vi "full_rt_layer.vi"() -> ()   [LabVIEW 2014]
uses:
  <vilib>/LabVIEW Targets/FPGA/cRIO/cRIO-9505/controls.llb/_nicrio_cRIO-9505_DriveStatus.ctl
  <vilib>/FPGAPlugInAG/cRIO-9074/niLvFpga_Open_cRIO-9074.vi
  <vilib>/Utility/error.llb/Error Cluster From Error Code.vi
  <vilib>/rvi/errors/niLvFpgaAdjustHostInterfaceError.vi
  <vilib>/FPGAPlugInAG/cRIO-9074/niLvFpga_Close_cRIO-9074.vi
  <vilib>/rvi/interface/nirviOpenFPGA/nirviOpenFPGA.xnode
  FPGA Bitfiles/MotorLabAProject_FPGATarget_fullfpgalayer_LolEBNhdJec.lvbitx
  full_fpga_layer.vi
  <vilib>/rvi/interface/nirviReadWriteControl/nirviReadWriteControl.xnode
  <vilib>/rvi/interface/nirviCloseFPGA/nirviCloseFPGA.xnode
  NiFpgaLv.dll
panel:
  out "PWM Current  Command":i16
  in  "number":i32
  out "Analog PID Scaled Output":fxp<+/-,34,17>
  in  "Reset Analog Counter":bool
  out "Set Point in Counts":dbl
  out "Waveform Chart 2":cluster{dbl, i32}(graph)
  out "Stepper Current (Steps)":i32
  out "Stepper Steps to move":i32
  in  "Reset Stepper Counter":bool
  out "PWM Angular Position":dbl
  out "Pot Angular \nPosition (deg)":fxp<+/-,33,11>
  out "error out":errorcluster
  in  "Position Loop  Rate (usec)":u16=250
  in  "Position Error Limit":i16=32767
  out "Position Error Read":i16
  out "Position Error Status":bool
  out "Encoder Position":i32
  in  "Reset Encoder Position":bool
  in  "stop":bool
  out "Drive Status":T1=enum."Disabled"
  out "Waveform Chart":cluster{i64, "PWM Encoder Position":i32}(graph)
  # "PWM SERVO"
  # "USE ESTOP!"
  # "ANALOG SERVO"
  # "STEPPER"
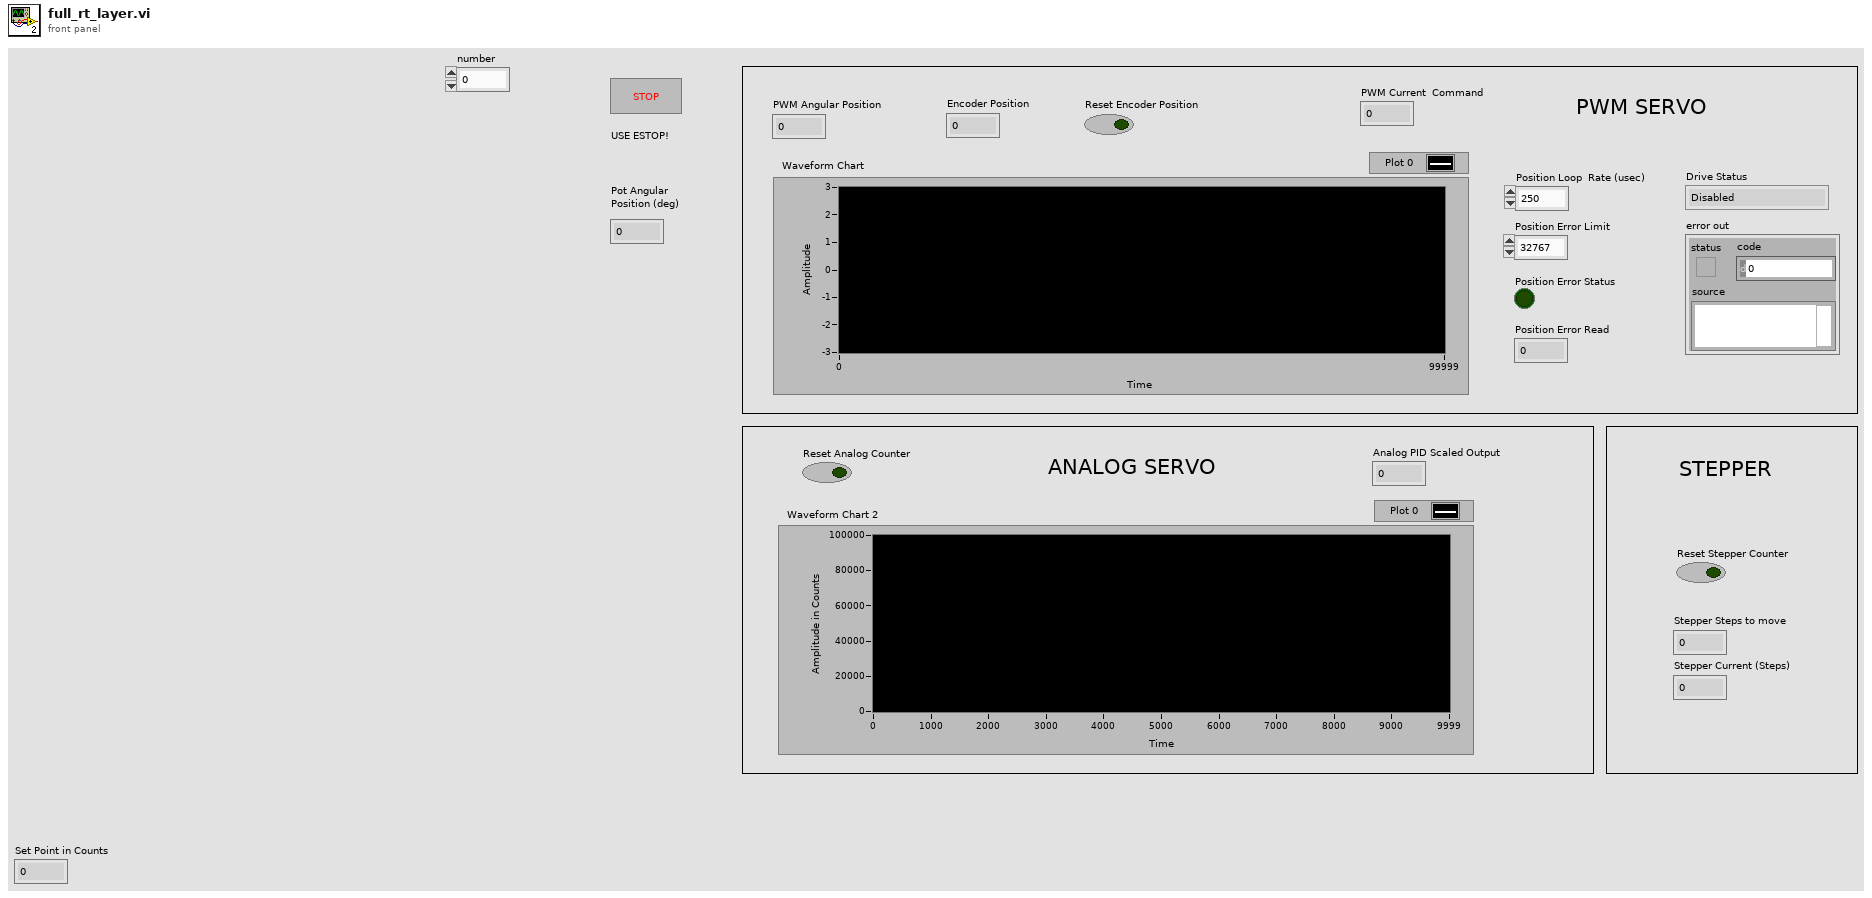
[diagram p1: front panel]
types:
  T1 = typedef "_nicrio_cRIO-9505_DriveStatus.ctl" = enum8{"Enabled", "Disabled", "Disabled by Drive Fault", "Disabled by Temp. Fault", "Disabled by E-Stop", "Unknown"}
  T2 = cluster{"Kp":i16, "Kd":i16, "Ki":i16, "ILim":i16, "Vff":i16, "Vff":i16, "Vff":i16, "Td":i16}
  T3 = cluster{dbl, "Analog Position  Feedback (Counts)":i32}
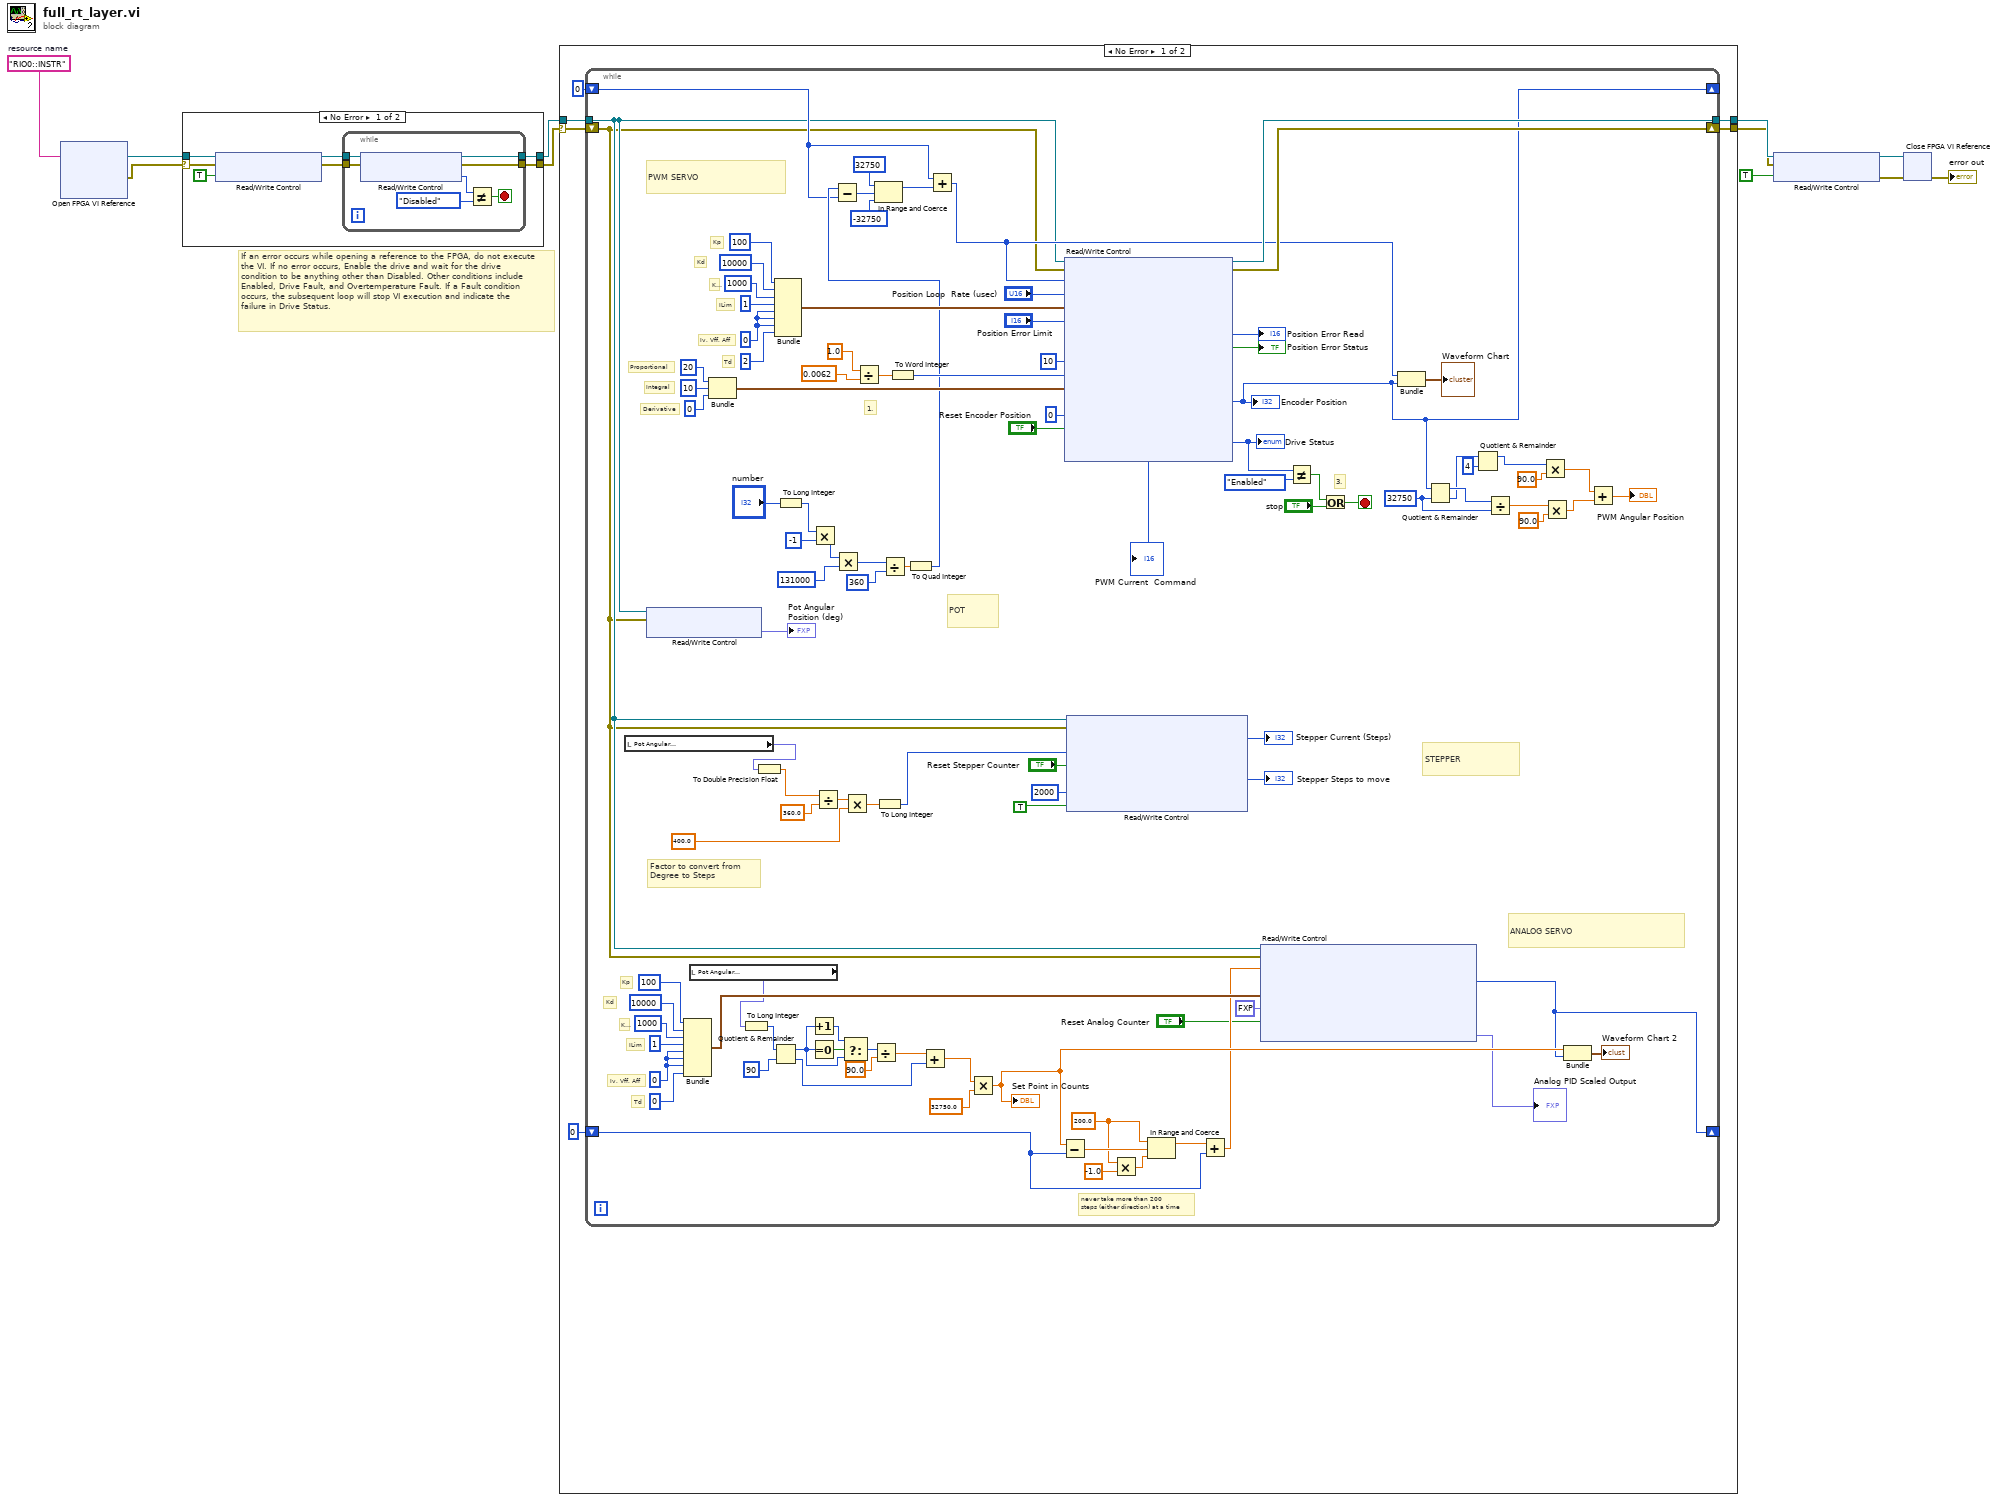
[diagram p0: block diagram]
diagram:
  w2 = "RIO0::INSTR"  # resource name
  # "If an error occurs while opening a reference to the FPGA, do not execute the VI. If no error occurs, Enable the drive and wait for the drive condition to be anything other than Disabled. Other conditions include Enabled, Drive Fault, and Overtemperature Fault. If a Fault condition occurs, the subsequent loop will stop VI execution and indicate the failure in Drive Status."
  n1 = xnode "Open FPGA VI Reference"("resource name"=w2) -> ("FPGA VI Reference Out"=w5:refnum<k20>, "error out"=w4:errorcluster)  [unwired: 1 in]
  n2 = case shown="No Error" w4 {
    selector: w4 -> [w13 w26]
    tunnel: w5 -> [w16 w27]
    tunnel: [w18 w27] -> w6
    tunnel: [w17 w26] -> w3
    frame No Error {
      n3 = xnode "Read/Write Control"("FPGA VI Reference In"=w16, "error in"=w13, "PWM  Enable Drive"=TRUE ("Enable Drive")) -> ("FPGA VI Reference Out"=w15:refnum<k20>, "error out"=w14:errorcluster)
      n4 = while {
        tunnel: [w25] -> w18
        tunnel: [w21] -> w17
        tunnel: w15 -> [w20]
        tunnel: w14 -> [w19]
        stop <- w22 stop-if-true
        n5 = xnode "Read/Write Control"("FPGA VI Reference In"=w20, "error in"=w19) -> ("FPGA VI Reference Out"=w25:refnum<k20>, "error out"=w21:errorcluster, "PWM Drive Status"=w24:T1)
        n6 = Not Equal?(x=w24, y=_nicrio_cRIO-9505_DriveStatus."Disabled") -> (x != y?=w22:bool)
      }
    }
    frame Error {
      # "Error occurred. Do not run."
    }
  }
  n7 = case shown="No Error" w3 {
    selector: w3 -> [w30 w139]
    tunnel: w6 -> [w33 w140]
    tunnel: [w32 w140] -> w11
    tunnel: [w31 w139] -> w10
    frame No Error {
      n8 = while {
        tunnel: w33 -> [w39]
        tunnel: [w134] -> w32
        shift-right: [w110] -> w31
        shift-left: w30 -> [w38]
        shift-right: [w89] -> _
        shift-left: 0 -> [w87]
        shift-right: [w42] -> _
        shift-left: 0 -> [w57]
        stop <- w111 stop-if-true
        w47 = 200.0
        w67 = i16 0 ("Vff")
        w108 = 32750 ("y")
        w120 = i16 0 ("Vff")
        # "never take more than 200 \nsteps (either direction) at a time"
        # "ANALOG SERVO"
        # "STEPPER"
        # "POT"
        # "Td"
        # "Iv, Vff, Aff"
        # "ILim"
        # "Ki"
        # "Kd"
        # "Kp"
        # "Factor to convert from \nDegree to Steps"
        # "PWM SERVO"
        # "Derivative"
        # "Integral"
        # "Proportional"
        # "Td"
        # "Iv, Vff, Aff"
        # "ILim"
        # "Ki"
        # "Kd"
        # "Kp"
        # "3."
        # "1."
        n9 = local read "Pot Angular \nPosition (deg)"() -> (w37:fxp<+/-,33,11>)
        n10 = xnode "Read/Write Control"("FPGA VI Reference In"=w39, "error in"=w38) -> ("Pot Angular Position"=→"Pot Angular \nPosition (deg)":fxp<+/-,33,11>)  [unwired: 2 out]
        n11 = Bundle("Kp"=i16 100, "Kd"=i16 10000, "Ki"=i16 1000, "ILim"=i16 1, "Vff"=w67, "Vff"=w67, "Vff"=w67, "Td"=i16 0) -> (w65:T2)  [unwired: 1 in]
        n12 = local read "Pot Angular \nPosition (deg)"() -> (w36:fxp<+/-,33,11>)
        n13 = Bundle("Td"=i16 20, "Td"=i16 10, "Td"=i16 0) -> (w114:cluster{"Td":i16, "Td":i16, "Td":i16})  [unwired: 1 in]
        n14 = To Long Integer(number=w36) -> (32bit integer=w41:i32)
        n15 = To Double Precision Float(number=w37) -> (double precision float=w51:dbl)
        n16 = Quotient & Remainder(x=w41, y=90) -> (x-y*floor(x/y)=w54:i32, floor(x/y)=w46:i32)
        n17 = Bundle("Kp"=i16 100, "Kd"=i16 10000, "Ki"=i16 1000, "ILim"=i16 1, "Vff"=w120, "Vff"=w120, "Vff"=w120, "Td"=i16 2) -> (w118:T2)  [unwired: 1 in]
        n18 = To Long Integer(number="number") -> (32bit integer=w86:i32)
        n19 = Increment(x=w54) -> (x+1=w53:i32)
        n20 = Equal To 0?(x=w54) -> (x = 0?=w55:bool)
        n21 = Multiply(x=w86, y=-1) -> (x*y=w85:i32)
        n22 = Divide(x=w51, y=360.0) -> (x/y=w83:dbl)
        n23 = Multiply(x=w85, y=131000) -> (x*y=w97:i32)
        n24 = Select(t=w53, s=w55, f=w54) -> (s? t:f=w52:i32)
        n25 = Multiply(x=w83, y=400.0) -> (x*y=w81:dbl)
        n26 = Divide(x=1.0, y=0.0062) -> (x/y=w130:dbl)
        n27 = Divide(x=w52, y=90.0) -> (x/y=w50:dbl)
        n28 = To Long Integer(number=w81) -> (32bit integer=w78:i32)
        n29 = Divide(x=w97, y=360) -> (x/y=w95:dbl)
        n30 = To Word Integer(number=w130) -> (16bit integer=w129:i16)
        n31 = To Quad Integer(1:w95) -> (0:w88:i64)
        n32 = Subtract(x=w88, y=w87) -> (x-y=w94:i64)
        n33 = In Range and Coerce(upper limit=i64 32750 ("lower limit"), x=w94, lower limit=i64 -32750) -> (coerced(x)=w91:i64)  [unwired: 1 out]
        n34 = Add(x=w50, y=w46) -> (x+y=w49:dbl)
        n35 = Add(x=w87, y=w91) -> (x+y=w90:i64)
        n36 = Multiply(x=w49, y=32750.0) -> (x*y=w48:dbl)
        "Set Point in Counts" <- w48
        n37 = Subtract(x=w48, y=w57) -> (x-y=w61:dbl)
        n38 = xnode "Read/Write Control"("FPGA VI Reference In"=w39, "error in"=w38, "PWM Position Setpoint"=w90, "PWM Position Loop  Rate (usec)"="Position Loop  Rate (usec)", "PWM Position PID Gains"=w118, "PWM Position Error Limit"="Position Error Limit", "PWM Current  Loop Rate (usec)"=u32 10, "PWM Current Limit"=w129, "PWM Current PI Gains"=w114, "PWM Reset Position Value"=0, "PWM Reset Position"="Reset Encoder Position") -> ("FPGA VI Reference Out"=w134:refnum<k20>, "error out"=w110:errorcluster, "PWM Position Error Read"=→"Position Error Read":i16, "PWM Position Error Status"=→"Position Error Status":bool, "PWM Encoder Position"=w89:i32, "PWM Drive Status"=w128:T1, "PWM Current  Command"=→"PWM Current  Command":i16)
        "Encoder Position" <- w89
        "Drive Status" <- w128
        n39 = xnode "Read/Write Control"("FPGA VI Reference In"=w39, "error in"=w38, "Stepper Desired Position (Steps)"=w78, "Stepper Reset Step Counter"="Reset Stepper Counter", "Stepper  Step Period (uS)"=i16 2000, "Stepper Enable/Disable Step Motor"=TRUE) -> ("Stepper Current (Steps)"=→"Stepper Current (Steps)":i32, "Stepper Steps to move"=→"Stepper Steps to move":i32)  [unwired: 2 out]
        n40 = Multiply(x=w47, y=-1.0) -> (x*y=w59:dbl)
        n41 = In Range and Coerce(upper limit=w47, x=w61, lower limit=w59) -> (coerced(x)=w58:dbl)  [unwired: 1 out]
        n42 = Add(x=w58, y=w57) -> (x+y=w45:dbl)
        n43 = xnode "Read/Write Control"("FPGA VI Reference In"=w39, "error in"=w38, "Analog Desired Position Setpoint (Counts)"=w45, "Analog PID Gains"=w65, "Analog Shutdown Signal"=fxp<+/-,20,5> 2.5, "Analog Reset Enc"="Reset Analog Counter") -> ("Analog Position  Feedback (Counts)"=w42:i32, "Analog PID Scaled Output"=→"Analog PID Scaled Output":fxp<+/-,34,17>)  [unwired: 2 out]
        n44 = Not Equal?(x=w128, y=_nicrio_cRIO-9505_DriveStatus."Enabled") -> (x != y?=w132:bool)
        n45 = Or(x=w132, y="stop") -> (x .or. y?=w111:bool)
        n46 = Bundle(w90, "PWM Encoder Position"=w89) -> (→"Waveform Chart":cluster{i64, "PWM Encoder Position":i32})  [unwired: 1 in]
        n47 = Quotient & Remainder(x=w89, y=w108) -> (x-y*floor(x/y)=w109:i32, floor(x/y)=w105:i32)
        n48 = Quotient & Remainder(x=w105, y=4) -> (x-y*floor(x/y)=w102:i32)  [unwired: 1 out]
        n49 = Divide(x=w109, y=w108) -> (x/y=w107:dbl)
        n50 = Multiply(x=w102, y=90.0) -> (x*y=w100:dbl)
        n51 = Multiply(x=w107, y=90.0) -> (x*y=w99:dbl)
        n52 = Bundle(w48, "Analog Position  Feedback (Counts)"=w42) -> (→"Waveform Chart 2":T3)  [unwired: 1 in]
        n53 = Add(x=w100, y=w99) -> (x+y=→"PWM Angular Position":dbl)
      }
    }
    frame Error {
      # "Error occurred. Do not run."
    }
  }
  n54 = xnode "Read/Write Control"("FPGA VI Reference In"=w11, "error in"=w10, "PWM Disable Drive"=TRUE ("Disable Drive")) -> ("FPGA VI Reference Out"=w9:refnum<k20>, "error out"=w8:errorcluster)
  n55 = xnode "Close FPGA VI Reference"("FPGA VI Reference In"=w9, "error in"=w8) -> ("error out"=→"error out":errorcluster)
